vi "Client - Launch Root Actor (Parrent).vi"(8 "error in":errorcluster) -> (0 "error out":errorcluster)   [LabVIEW 2023, in "Client.lvlib" / "Client.lvclass"]
uses:
  Client.lvclass
  <vilib>/ActorFramework/Actor/Actor.lvclass
  Parent/Parent_Class.lvclass
  Client - Ctrl - FGV - Action.ctl
panel:
  # "LAUNCHER"
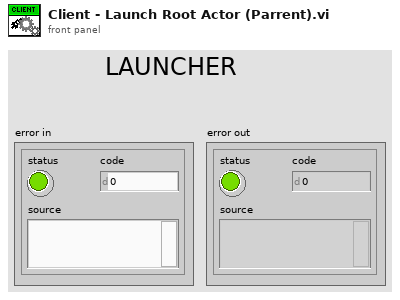
[diagram p1: front panel]
types:
  T1 = typedef "Client.lvlib/Client.lvclass/Client - Ctrl - FGV - Action.ctl" = enum16{"Int", "Get"}
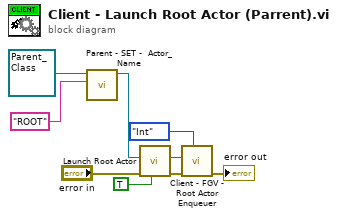
[diagram p0: block diagram]
diagram:
  n1 = call "Parent - SET -  Actor_Name.vi"("Actor_Name"="ROOT", "Parent_Class in"=refnum<class "Parent_Class.lvclass"> refnum ("Actor_Parent.lvlib:Parent_Class.lvclass")) -> ("Parent_Class out"=w2:refnum<class "Parent_Class.lvclass">)  [unwired: 8 in, 1 out]
  n2 = call <vilib>:"Launch Root Actor.vi"("Open Actor Core front panel? (F)"=TRUE, "error in (no error)"="error in", "Actor"=w2) -> ("error out"=w8:errorcluster, "Actor's Enqueuer"=w7:refnum<class "Message Enqueuer.lvclass">)  [unwired: 7 in]
  n3 = call "Client - FGV - Root Actor Enqueuer.vi"("Action"=Client_-_Ctrl_-_FGV_-_Action."Int", "error in"=w8, "Actor's Enqueuer"=w7) -> ("error out"=→"error out":errorcluster)  [unwired: 7 in, 1 out]
